vi "导电机制拟合.vi"(8 "数据":dbl[][](array[numeric])) -> ()   [LabVIEW 2020]
uses:
  <vilib>/Analysis/NI_AALPro.lvlib
panel:
  out "XY图":cluster{dbl[], dbl[]}[](graph)
  out "字符串":string
  in  "映射方式":T1
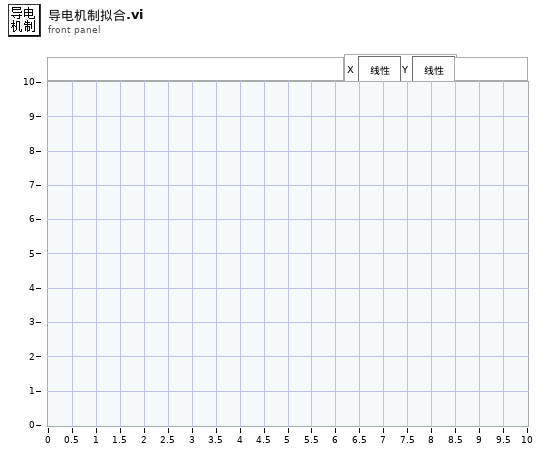
[diagram p1: front panel]
types:
  T1 = typedef "数据显示.xctl/映射方式.ctl" = cluster{"X":bool, "Y":bool}
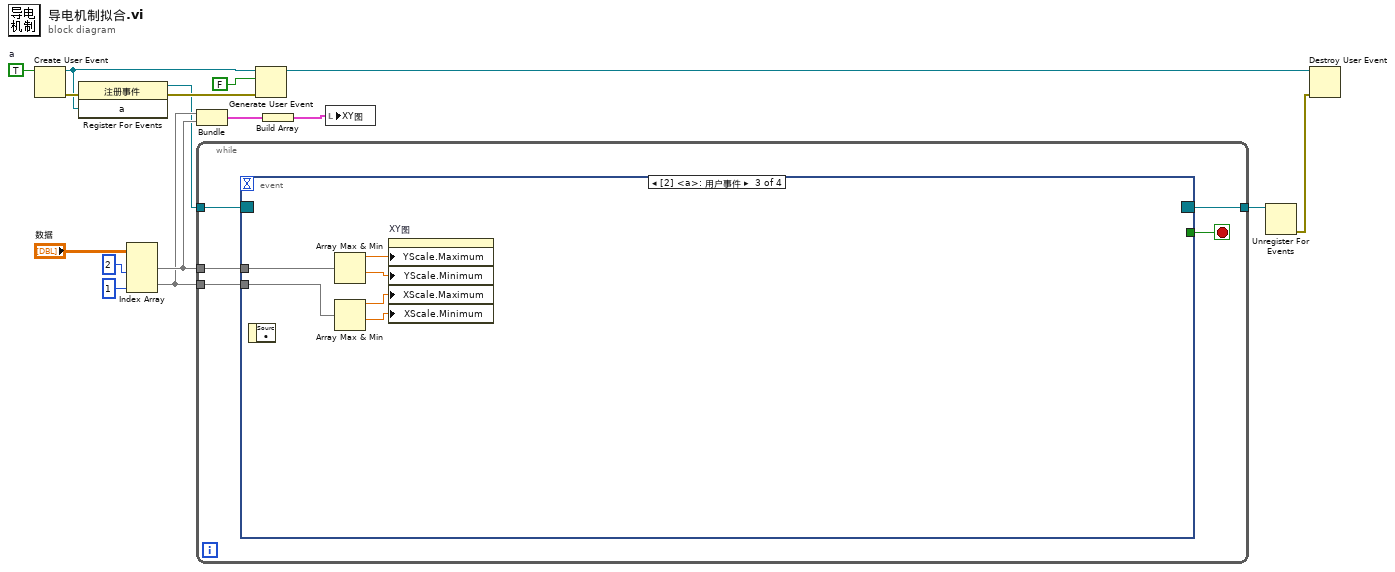
[diagram p0: block diagram]
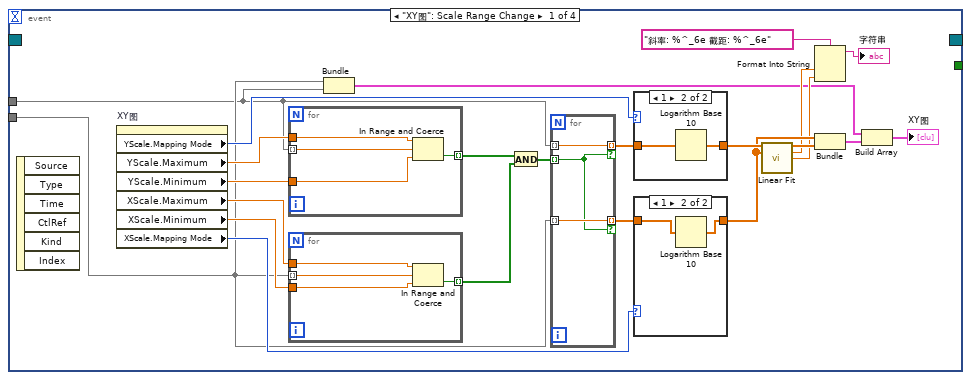
[diagram p2: hidden frame]
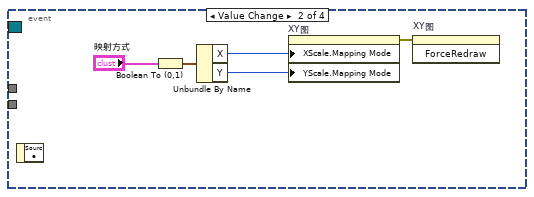
[diagram p5: hidden frame]
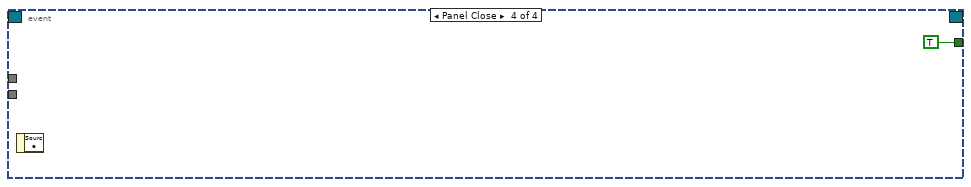
[diagram p6: hidden frame]
diagram:
  w9 = TRUE  # a
  n1 = Create User Event(user event datatype=w9) -> (user event=w7:refnum<user-event>, error out=w8:errorcluster)  [unwired: 1 in]
  n2 = register-events(error in=w8, w7) -> (reference out=w4:refnum<event-registration>, error out=w6:errorcluster)  [unwired: 1 in]
  n3 = Index Array(array="数据", index (col) #1=2 ("禁用的索引 (列)"), index (col) #2=1 ("索引 (列)")) -> (element #1=w12:dbl[], element #2=w11:dbl[])  [unwired: 2 in]
  n4 = Bundle("数据"=w11, "数据"=w12) -> (w16:cluster{"数据":dbl[], "数据":dbl[]})  [unwired: 1 in]
  n5 = while {
    tunnel: w11 -> [w21]
    tunnel: w12 -> [w20]
    tunnel: w4 -> [w18]
    tunnel: [w17] -> w3
    stop <- w19 stop-if-true
    n6 = event shown="[2] <a>: 用户事件" {
      selector: w18 -> [_ _ _ _]
      dyn-events: [_ _ _ _] -> w17
      timeout: _ -> [_ _ _ _]
      tunnel: w21 -> [w26 _ w69 _]
      tunnel: w20 -> [w25 _ w72 _]
      tunnel: [_ _ _ TRUE] -> w19
      event "XY图": Scale Range Change {
        n7 = event-data() -> ()  [unwired: 1 in, 6 out]
        n8 = property on="XY图" class="XYGraph (严格)"() -> ("YScale.Mapping Mode"=w40:u8, "YScale.Maximum"=w37:dbl, "YScale.Minimum"=w36:dbl, "XScale.Maximum"=w35:dbl, "XScale.Minimum"=w34:dbl, "XScale.Mapping Mode"=w33:u8)  [unwired: 2 in, 2 out]
        n9 = for {
          tunnel: w25 -> [w55] mode=indexing
          tunnel: w37 -> [w57]
          tunnel: w36 -> [w56]
          tunnel: [w54] -> w38 mode=indexing
          n10 = In Range and Coerce(upper limit=w57, x=w55, lower limit=w56) -> (In Range?=w54:bool)  [unwired: 1 out]
        }
        n11 = for {
          tunnel: w26 -> [w59] mode=indexing
          tunnel: w35 -> [w61]
          tunnel: w34 -> [w60]
          tunnel: [w58] -> w39 mode=indexing
          n12 = In Range and Coerce(upper limit=w61, x=w59, lower limit=w60) -> (In Range?=w58:bool)  [unwired: 1 out]
        }
        n13 = Bundle("数据"=w26, "数据"=w25) -> (w24:cluster{"数据":dbl[], "数据":dbl[]})  [unwired: 1 in]
        n14 = And(x=w38, y=w39) -> (x .and. y?=w44:bool[])
        n15 = for {
          tunnel: w44 -> [w51] mode=indexing
          tunnel: w26 -> [w53] mode=indexing
          tunnel: w25 -> [w52] mode=indexing
          tunnel: [w53] -> w43 mode=indexing if=w51
          tunnel: [w52] -> w42 mode=indexing if=w51
        }
        n16 = case shown="1" w40 {
          tunnel: w42 -> [w45 w47]
          tunnel: [w45 w46] -> w41
          frame 0, Default {
          }
          frame 1 {
            n17 = Logarithm Base 10(1:w47) -> (0:w46:dbl[])
          }
        }
        n18 = case shown="1" w33 {
          tunnel: w43 -> [w48 w50]
          tunnel: [w48 w49] -> w32
          frame 0, Default {
          }
          frame 1 {
            n19 = Logarithm Base 10(1:w50) -> (0:w49:dbl[])
          }
        }
        n20 = call <vilib>:"Linear Fit.vi"("Y"=w41, "X"=w32) -> ("Best Linear Fit"=w31:dbl[], "slope"=w28:dbl, "intercept"=w27:dbl)  [unwired: 9 in, 2 out]
        n21 = Format Into String(format string="斜率: %^_6e 截距: %^_6e" ("格式字符串"), w28, w27) -> (resulting string=→"字符串":string)  [unwired: 2 in, 1 out]
        n22 = Bundle(w32, "Best Linear Fit"=w31) -> (w30:cluster{dbl[], "Best Linear Fit":dbl[]})  [unwired: 1 in]
        n23 = Build Array(w24, w30) -> (→"XY图":cluster{"数据":dbl[], "Best Linear Fit":dbl[]}[])
      }
      event Value Change {
        n24 = event-data() -> ()  [unwired: 1 in, 1 out]
        n25 = Boolean To (0,1)(Boolean="映射方式") -> (0, 1=w65:cluster{"X":i16, "Y":i16})
        n26 = Unbundle By Name(w65) -> ("X"=w64:i16, "Y"=w63:i16)
        n27 = property on="XY图" class="XYGraph (严格)"("XScale.Mapping Mode"=w64, "YScale.Mapping Mode"=w63) -> (error out=w62:errorcluster)  [unwired: 2 in, 1 out]
        n28 = invoke on="XY图" class="XYGraph (严格)" method="ForceRedraw"(error in=w62) -> ()  [unwired: 2 in, 3 out]
      }
      event User Event {
        n29 = event-data() -> ()  [unwired: 1 in, 1 out]
        n30 = Array Max & Min(array=w72) -> (max value=w71:dbl, min value=w70:dbl)  [unwired: 2 out]
        n31 = Array Max & Min(array=w69) -> (max value=w68:dbl, min value=w67:dbl)  [unwired: 2 out]
        n32 = property on="XY图" class="XYGraph (严格)"("YScale.Maximum"=w71, "YScale.Minimum"=w70, "XScale.Maximum"=w68, "XScale.Minimum"=w67) -> ()  [unwired: 2 in, 2 out]
      }
      event Panel Close {
        n33 = event-data() -> ()  [unwired: 1 in, 1 out]
      }
    }
  }
  n34 = Generate User Event(user event=w7, event data cluster=FALSE ("事件数据"), error in=w6) -> (user event out=w2:refnum<user-event>)  [unwired: 1 in, 1 out]
  n35 = Build Array(w16) -> (w10:cluster{"数据":dbl[], "数据":dbl[]}[])
  n36 = local write "XY图"(w10) -> ()
  n37 = Unregister For Events(event registration refnum=w3) -> (error out=w1:errorcluster)  [unwired: 1 in]
  n38 = Destroy User Event(user event=w2, error in=w1) -> ()  [unwired: 1 out]
